vi "Get Value STR.vi"(0 "Session Handle in":T1, 5 "Lookup String":string, 11 "error in (no error)":errorcluster) -> (4 "Session Handle out":T1, 6 "Value":string, 15 "error out":errorcluster)   [LabVIEW 2019, in "HTS.lvlib" / "VariableContainer.lvclass"]
uses:
  VariableContainer.lvclass
  Typedefs/Session Handle.ctl
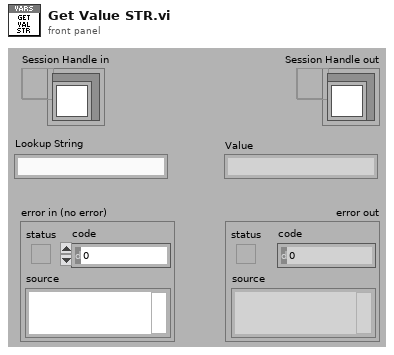
[diagram p1: front panel]
types:
  T1 = typedef "HTS.lvlib/VariableContainer.lvclass/Session Handle.ctl" = refnum<data-value>
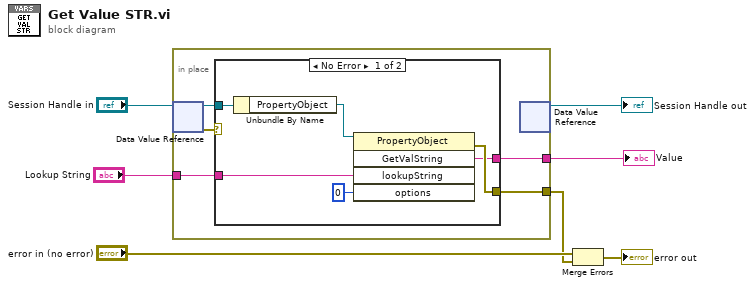
[diagram p0: block diagram]
diagram:
  n1 = in-place {
    in-place-border: "Lookup String" -> [w10]
    in-place-border: [w9] -> w4
    in-place-border: [w8] -> w1
    n2 = in-place-dvr #1("Session Handle in") -> (w12:refnum<class "VariableContainer.lvclass">, w11:errorcluster)
    n3 = case shown="No Error" w11 {
      selector: w11 -> [_ w19]
      tunnel: w12 -> [w17 _]
      tunnel: w10 -> [w15 _]
      tunnel: [w13 _] -> w9
      tunnel: [w18 w19] -> w8
      frame No Error {
        n4 = Unbundle By Name(w17) -> ("PropertyObject"=w16:refnum<k7>)
        n5 = invoke class="PropertyObject" method="GetValString"(reference=w16, "lookupString"=w15, "options"=0) -> (error out=w18:errorcluster, "GetValString"=w13:string)  [unwired: 2 in, 3 out]
      }
      frame Error {
      }
    }
    n6 = in-place-dvr #1() -> (→"Session Handle out":T1)  [unwired: 1 in, 1 out]
  }
  "Value" <- w4
  n7 = Merge Errors("error in (no error)", w1) -> (→"error out":errorcluster)
